vi "strain_correcter.vi"(1 "raw max":dbl=0.002 format="%#_13g", 2 "raw normal":dbl=0.000650527 format="%#_13g", 3 "raw min":dbl=-0.0009067 format="%#_13g", 5 "max":dbl, 7 "min":dbl, 9 "normal":dbl=1.0, 11 "Raw strain":dbl) -> (8 "strain":dbl)   [LabVIEW 2022 SP3]
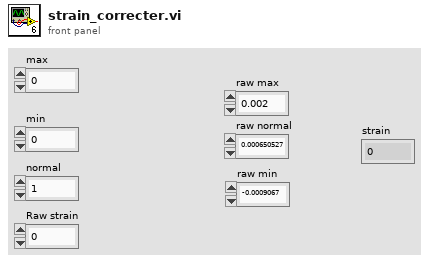
[diagram p1: front panel]
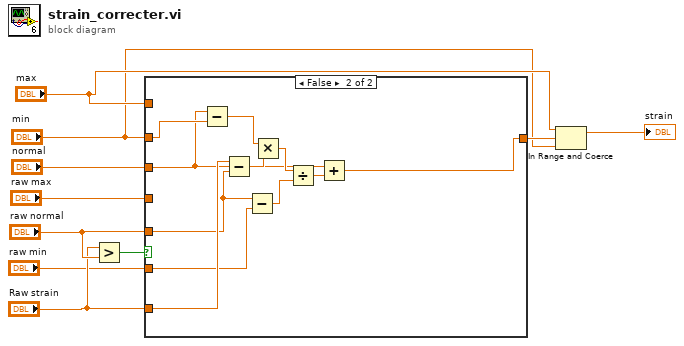
[diagram p0: block diagram]
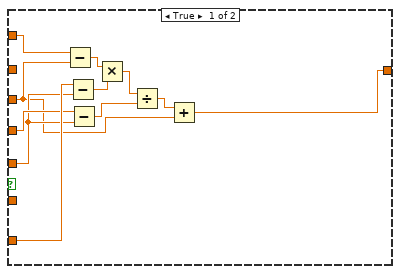
[diagram p2: hidden frame]
diagram:
  n1 = Greater?(x="Raw strain", y="raw normal") -> (0:w10:bool)
  n2 = case shown="False" w10 {
    tunnel: "raw normal" -> [w18 w26]
    tunnel: "Raw strain" -> [w20 w28]
    tunnel: "raw max" -> [w19 _]
    tunnel: "max" -> [w21 _]
    tunnel: [w11 w22] -> w4
    tunnel: "raw min" -> [_ w25]
    tunnel: "min" -> [_ w27]
    tunnel: "normal" -> [w12 w23]
    frame True {
      n3 = Subtract(x=w21, y=w12) -> (x-y=w17:dbl)
      n4 = Subtract(x=w20, y=w18) -> (x-y=w16:dbl)
      n5 = Subtract(x=w19, y=w18) -> (x-y=w14:dbl)
      n6 = Multiply(x=w17, y=w16) -> (x*y=w15:dbl)
      n7 = Divide(x=w15, y=w14) -> (x/y=w13:dbl)
      n8 = Add(x=w13, y=w12) -> (x+y=w11:dbl)
    }
    frame False {
      n9 = Subtract(x=w23, y=w27) -> (x-y=w32:dbl)
      n10 = Subtract(x=w28, y=w26) -> (x-y=w31:dbl)
      n11 = Subtract(x=w26, y=w25) -> (x-y=w29:dbl)
      n12 = Multiply(x=w32, y=w31) -> (x*y=w30:dbl)
      n13 = Divide(x=w30, y=w29) -> (x/y=w24:dbl)
      n14 = Add(x=w23, y=w24) -> (x+y=w22:dbl)
    }
  }
  n15 = In Range and Coerce(upper limit="max", x=w4, lower limit="min") -> (coerced(x)=→"strain":dbl)  [unwired: 1 out]
